vi "Fetch records from DB.vi"(4 "error in":errorcluster, 7 "Query":string) -> (0 "error out":errorcluster, 3 "recordset data":variant[][](array[variant]))   [LabVIEW 2010]
uses:
  <vilib>/addons/database/Connection.llb/DB Tools Open Connec (Path).vi
  <vilib>/addons/database/Connection.llb/Conn Execute.vi
  <vilib>/addons/database/Recordset.llb/Rec Fetch Recordset Data (R).vi
  <vilib>/addons/database/Recordset.llb/Rec Destroy - Connection.vi
  <vilib>/addons/database/NI_Database_API.lvlib
panel:
  out "Array 3":variant[][](array[variant])
  out "Array 2":string[][](array[string])
  out "Array":string[](array[string])
  out "type string":i16[][](array[numeric]) format="%04x"
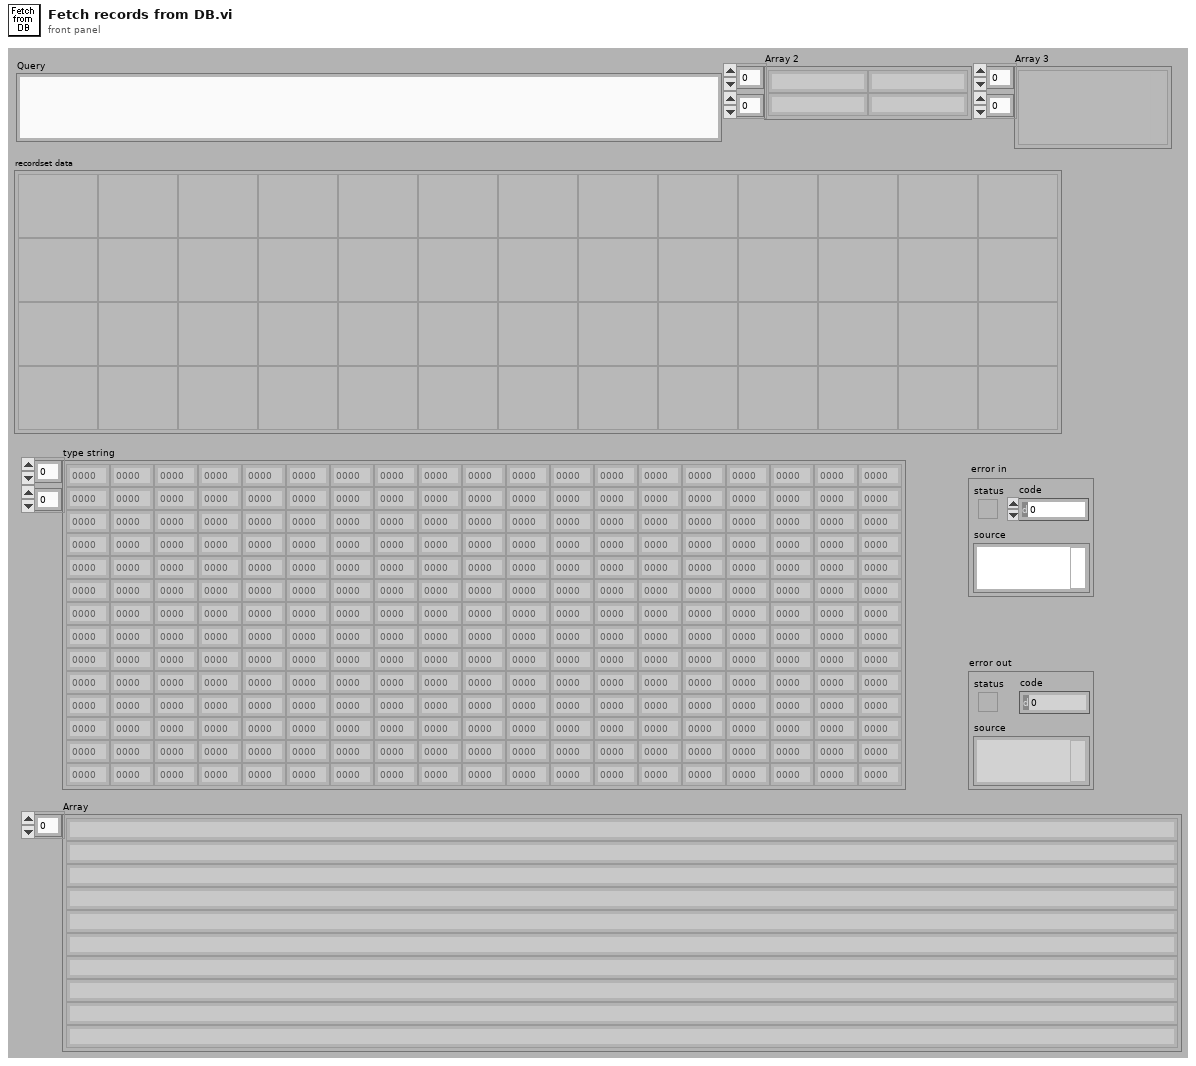
[diagram p1: front panel]
types:
  T1 = typedef "NI_Database_API.lvlib/Conn ObjectReference.ctl" = refnum<k1>
  T2 = typedef "NI_Database_API.lvlib/Rec ObjectReference.ctl" = refnum<k1>
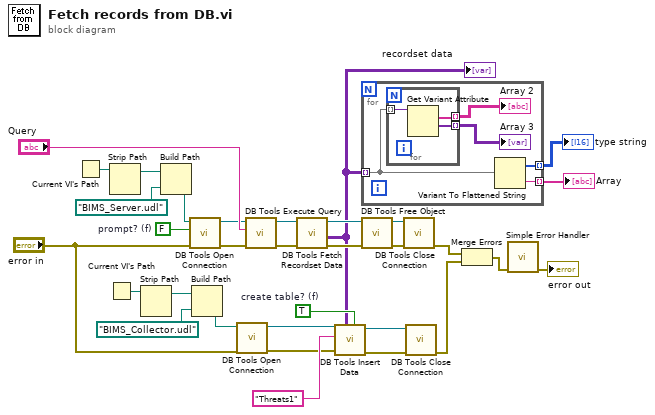
[diagram p0: block diagram]
diagram:
  w11 = TRUE  # create table? (f)
  w23 = FALSE  # prompt? (f)
  n1 = Current VI's Path() -> (path=w20:path)
  n2 = Current VI's Path() -> (path=w14:path)
  n3 = Strip Path(path=w20) -> (stripped path=w21:path)  [unwired: 1 out]
  n4 = Strip Path(path=w14) -> (stripped path=w17:path)  [unwired: 1 out]
  n5 = Build Path(base path=w21, name or relative path=path "BIMS_Server.udl" ("Application:Directory Path")) -> (appended path=w19:path)
  n6 = call-poly <vilib>:"DB Tools Open Connection.vi"("error in (no error)"="error in", "prompt? (F)"=w23, "connection information"=w19) -> ("error out"=w31:errorcluster, "connection reference"=w24:T1)  [unwired: 2 in, 3 out]
  n7 = Build Path(base path=w17, name or relative path=path "BIMS_Collector.udl" ("Application:Directory Path")) -> (appended path=w16:path)
  n8 = call-poly <vilib>:"DB Tools Open Connection.vi"("error in (no error)"="error in", "connection information"=w16) -> ("error out"=w9:errorcluster, "connection reference"=w15:T1)  [unwired: 3 in, 3 out]
  n9 = call-poly <vilib>:"DB Tools Execute Query.vi"("error in (no error)"=w31, "SQL query"="Query", "connection reference"=w24) -> ("error out"=w30:errorcluster, "recordset reference"=w25:T2)  [unwired: 1 in, 4 out]
  n10 = call-poly <vilib>:"DB Tools Fetch Recordset Data.vi"("error in (no error)"=w30, "recordset reference"=w25) -> ("error out"=w29:errorcluster, "recordset data"=w3:variant[][], "recordset reference out"=w26:T2)  [unwired: 3 out]
  "recordset data" <- w3
  n11 = call <vilib>:"DB Tools Insert Data.vi"("create table? (F)"=w11, "data"=w3, "error in (no error)"=w9, "table"="Threats1" ("Query"), "connection reference"=w15) -> ("error out"=w7:errorcluster, "connection reference out"=w8:T1)  [unwired: 2 in, 3 out]
  n12 = for {
    tunnel: w3 -> [w35] mode=indexing
    tunnel: [w37] -> w2 mode=indexing
    tunnel: [w36] -> w1 mode=indexing
    n13 = for {
      tunnel: w35 -> [w39] mode=indexing
      tunnel: [w40] -> w34 mode=indexing
      tunnel: [w38] -> w33 mode=indexing
      n14 = Get Variant Attribute(Variant=w39) -> (names=w40:string[], values=w38:variant[])  [unwired: 1 in, 4 out]
    }
    "Array 2" <- w34
    "Array 3" <- w33
    n15 = Variant To Flattened String(Variant=w35) -> (data string=w36:string, 1:w37:i16[])
  }
  "type string" <- w2
  "Array" <- w1
  n16 = call-poly <vilib>:"DB Tools Free Object.vi"("error in (no error)"=w29, "recordset reference"=w26) -> ("error out"=w28:errorcluster, "connection reference"=w27:T1)  [unwired: 8 out]
  n17 = call <vilib>:"DB Tools Close Connection.vi"("error in (no error)"=w28, "connection reference"=w27) -> ("error out"=w6:errorcluster)  [unwired: 5 out]
  n18 = call <vilib>:"DB Tools Close Connection.vi"("error in (no error)"=w7, "connection reference"=w8) -> ("error out"=w5:errorcluster)  [unwired: 5 out]
  n19 = Merge Errors(w6, w5) -> (w4:errorcluster)
  n20 = call <vilib>:"Simple Error Handler.vi"("error in (no error)"=w4) -> ("error out"=→"error out":errorcluster)  [unwired: 1 in, 7 out]
